vi "IndustrialReadCustomRule.vi"(11 "Custom Rule":string) -> (3 "IsImmediate":bool)   [LabVIEW 2020, in "NI_Variable.lvlib"]
uses:
  <vilib>/variable/NI_Variable.lvlib
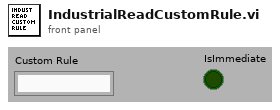
[diagram p1: front panel]
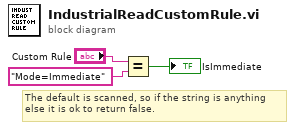
[diagram p0: block diagram]
diagram:
  # "The default is scanned, so if the string is anything\nelse it is ok to return false."
  n1 = Equal?(x="Custom Rule", y="Mode=Immediate" ("regular expression")) -> (x = y?=→"IsImmediate":bool)
